vi "Begin.vi"() -> (0 "error out":errorcluster)   [LabVIEW 2013]
doc: "Called before other user functions, this VI is expected to open initial I/O refnums, load in file data, and do all program initialization. Notice that the <B>error out</B> terminal is simply used for data flow. Wiring it to other structures or subVIs ensures that this VI runs first."
uses:
  <vilib>/Rock Robotics/WPI/DriverStation/WPI_DriverStationRobotMode2.ctl
  <vilib>/Rock Robotics/WPI/Joystick/WPI_JoystickDeviceEnum.ctl
  <vilib>/Rock Robotics/SystemInterfaces/DIO/FPGA_DIOPWMChannel.ctl
  <vilib>/Rock Robotics/WPI/SafetyOutput/WPI_SafetyOutputConfigMenu.ctl
  Robot Global Data.vi
  <vilib>/Rock Robotics/WPI/RobotDrive/WPI_RobotDriveOpen4MotorWithJaguar.vi
  <vilib>/Rock Robotics/WPI/MotorControl/WPI_MotorControlOpen Jaguar.vi
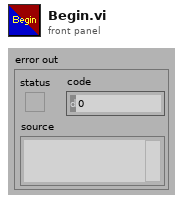
[diagram p1: front panel]
types:
  T1 = typedef "FPGA_DIOPWMChannel.ctl" = enum8{"PWM 1", "PWM 2", "PWM 3", "PWM 4", "PWM 5", "PWM 6", "PWM 7", "PWM 8", "PWM 9", "PWM 10", "Invalid"}
  T2 = typedef "WPI_SafetyOutputConfigMenu.ctl" = enum16{"Enable", "Disable"}
  T3 = typedef "WPI_JoystickDeviceEnum.ctl" = enum16{"USB 1", "USB 2", "USB 3", "USB 4", "Kinect 1", "Kinect 2"}
  T4 = typedef "WPI_DriverStationRobotMode2.ctl" = enum16{"Autonomous Disabled", "Autonomous Enabled", "Teleop Disabled", "Teleop Enabled", "Timeout", "Finish", "Test Disabled", "Test Enabled"}
  T5 = typedef "WPI_JoystickDevRef.ctl" = cluster{"Device":T3}
  T6 = typedef "WPI_MotorControlDeviceRef.ctl" = cluster{"DeviceStatus":errorcluster, "Type":enum16{"PWM", "CAN"}, "PWM":cluster{"Digital Module":T7, "PWM Channel":T1, "DeadBand":T8}, "CAN":cluster{"Device Number":u8, "Control Mode":T9, "Semaphore":T10, "Max Vout":dbl}, "Invert":bool, "TransformRef":T11, "InvTransformRef":T11}
  T7 = typedef "FPGA_TypedefDigitalModule.ctl" = enum16{"Digital Module 1", "Digital Module 2"}
  T8 = typedef "WPI_PWMDeadband.ctl" = cluster{"Name":string, "maxPositivePwm":i32, "minPositivePwm":i32, "centerPwm":i32, "maxNegativePwm":i32, "minNegativePwm":i32, "angularRange":u16}
  T9 = typedef "WPI_CANJaguar_ControlMode.ctl" = enum8{"Percent VBus", "Current", "Speed", "Position", "Voltage"}
  T10 = typedef "Semaphore RefNum" = refnum<k1>
  T11 = typedef "WPI_PWMTransform_ConPane.ctl" = refnum<vi>
  T12 = typedef "WPI_RobotDriveDevRef.ctl" = cluster{"DevStatus":errorcluster, "Motors[]":T6[], "Square Inputs":bool, "Max Output":dbl, "Isochronous":bool}
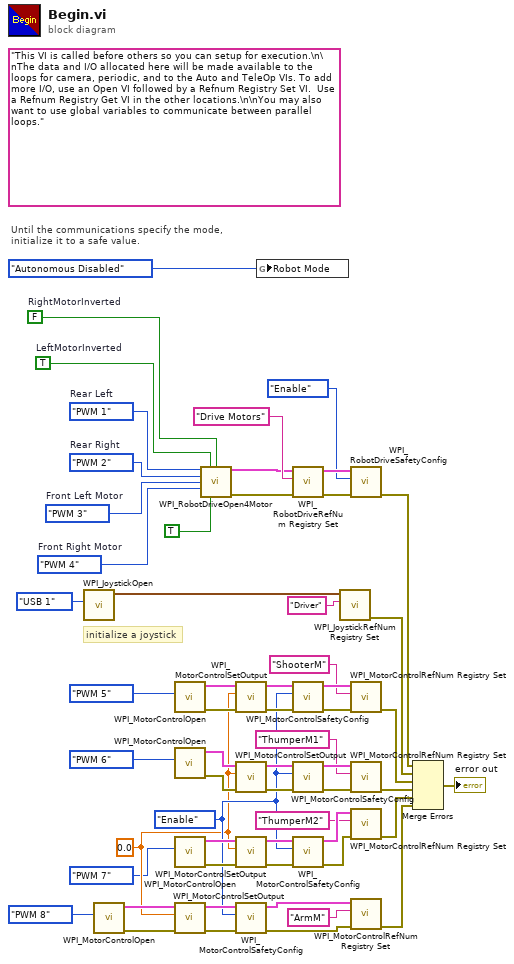
[diagram p0: block diagram]
diagram:
  w13 = 0.0 ("Output")
  w14 = WPI_SafetyOutputConfigMenu."Enable" ("mode")
  w45 = FPGA_DIOPWMChannel."PWM 4"  # Front Right Motor
  w46 = FPGA_DIOPWMChannel."PWM 3"  # Front Left Motor
  w49 = FPGA_DIOPWMChannel."PWM 2"  # Rear Right
  w50 = FPGA_DIOPWMChannel."PWM 1"  # Rear Left
  w53 = TRUE  # LeftMotorInverted
  w54 = FALSE  # RightMotorInverted
  (unwired) "This VI is called before others so you can setup for execution.\n\nThe data and I/O allocated here will be made available to the loops for camera, periodic, and to the Auto and TeleOp VIs. To add more I/O, use an Open VI followed by a Refnum Registry Set VI.  Use a Refnum Registry Get VI in the other locations.\n\nYou may also want to use global variables to communicate between parallel loops."
  # "initialize a joystick"
  # "Until the communications specify the mode,\ninitialize it to a safe value."
  n1 = call <vilib>:"WPI_JoystickOpen.vi"("JoystickDevice"=WPI_JoystickDeviceEnum."USB 1") -> ("JoystickDevRef"=w56:T5)  [unwired: 10 in]
  n2 = call-poly <vilib>:"WPI_MotorControlOpen.vi"("PWM Channel"=FPGA_DIOPWMChannel."PWM 8") -> ("error out"=w24:errorcluster, "MotorControlDeviceRef"=w25:T6)  [unwired: 9 in]
  n3 = call-poly <vilib>:"WPI_MotorControlOpen.vi"("PWM Channel"=FPGA_DIOPWMChannel."PWM 5") -> ("error out"=w15:errorcluster, "MotorControlDeviceRef"=w29:T6)  [unwired: 9 in]
  n4 = call-poly <vilib>:"WPI_MotorControlOpen.vi"("PWM Channel"=FPGA_DIOPWMChannel."PWM 6") -> ("error out"=w28:errorcluster, "MotorControlDeviceRef"=w30:T6)  [unwired: 9 in]
  n5 = call-poly <vilib>:"WPI_MotorControlOpen.vi"("PWM Channel"=FPGA_DIOPWMChannel."PWM 7") -> ("error out"=w26:errorcluster, "MotorControlDeviceRef"=w27:T6)  [unwired: 9 in]
  n6 = call <vilib>:"WPI_MotorControlSetOutput.vi"("error in (no error)"=w24, "Output"=w13, "MotorControlDevRef"=w25) -> ("error out"=w23:errorcluster, "MotorControlDevRef"=w22:T6)  [unwired: 6 in, 1 out]
  n7 = call-poly <vilib>:"WPI_RobotDriveOpen4Motor.vi"("Rear Left Motor"=w50, "Rear Left Motor Inverted"=w53, "Rear Right Motor Inverted"=w54, "Rear Right Motor"=w49, "Front Left Motor"=w46, "Front Right Motor"=w45, "Front Left Motor Inverted"=TRUE) -> ("RobotDriveDevRef"=w42:T12, "error out"=w51:errorcluster)  [unwired: 7 in]
  n8 = call <vilib>:"WPI_MotorControlSetOutput.vi"("error in (no error)"=w15, "Output"=w13, "MotorControlDevRef"=w29) -> ("error out"=w16:errorcluster, "MotorControlDevRef"=w17:T6)  [unwired: 6 in, 1 out]
  n9 = call <vilib>:"WPI_MotorControlSetOutput.vi"("error in (no error)"=w28, "Output"=w13, "MotorControlDevRef"=w30) -> ("error out"=w18:errorcluster, "MotorControlDevRef"=w19:T6)  [unwired: 6 in, 1 out]
  n10 = call <vilib>:"WPI_MotorControlSetOutput.vi"("error in (no error)"=w26, "Output"=w13, "MotorControlDevRef"=w27) -> ("error out"=w20:errorcluster, "MotorControlDevRef"=w21:T6)  [unwired: 6 in, 1 out]
  n11 = call <vilib>:"WPI_MotorControlSafetyConfig.vi"("error in (no error)"=w23, "mode"=w14, "MotorControlDevRef"=w22) -> ("error out"=w35:errorcluster, "MotorControlDevRef"=w36:T6)  [unwired: 7 in]
  n12 = global write "Robot Global Data.vi" "Robot Mode"(WPI_DriverStationRobotMode2."Autonomous Disabled" ("Robot Mode")) -> ()
  n13 = call <vilib>:"WPI_RobotDriveRefNum Registry Set.vi"("error in (no error)"=w51, "refnum name"="Drive Motors", "RobotDriveDevRef"=w42) -> ("error out"=w43:errorcluster, "RobotDriveDevRef"=w48:T12)  [unwired: 7 out]
  n14 = call <vilib>:"WPI_MotorControlSafetyConfig.vi"("error in (no error)"=w16, "mode"=w14, "MotorControlDevRef"=w17) -> ("error out"=w32:errorcluster, "MotorControlDevRef"=w33:T6)  [unwired: 7 in]
  n15 = call <vilib>:"WPI_MotorControlSafetyConfig.vi"("error in (no error)"=w18, "mode"=w14, "MotorControlDevRef"=w19) -> ("error out"=w31:errorcluster, "MotorControlDevRef"=w34:T6)  [unwired: 7 in]
  n16 = call <vilib>:"WPI_MotorControlSafetyConfig.vi"("error in (no error)"=w20, "mode"=w14, "MotorControlDevRef"=w21) -> ("error out"=w37:errorcluster, "MotorControlDevRef"=w38:T6)  [unwired: 7 in]
  n17 = call <vilib>:"WPI_JoystickRefNum Registry Set.vi"("refnum name"="Driver", "JoystickDevRef"=w56) -> ("error out"=w39:errorcluster)  [unwired: 8 in, 1 out]
  n18 = call <vilib>:"WPI_RobotDriveSafetyConfig.vi"("error in (no error)"=w43, "mode"=WPI_SafetyOutputConfigMenu."Enable", "RobotDriveDevRef"=w48) -> ("error out"=w40:errorcluster)  [unwired: 7 in, 1 out]
  n19 = call <vilib>:"WPI_MotorControlRefNum Registry Set.vi"("error in (no error)"=w32, "refnum name"="ShooterM", "MotorControlDevRef"=w33) -> ("error out"=w8:errorcluster)  [unwired: 7 in, 1 out]
  n20 = call <vilib>:"WPI_MotorControlRefNum Registry Set.vi"("error in (no error)"=w31, "refnum name"="ThumperM1", "MotorControlDevRef"=w34) -> ("error out"=w7:errorcluster)  [unwired: 7 in, 1 out]
  n21 = call <vilib>:"WPI_MotorControlRefNum Registry Set.vi"("error in (no error)"=w37, "refnum name"="ThumperM2", "MotorControlDevRef"=w38) -> ("error out"=w6:errorcluster)  [unwired: 7 in, 1 out]
  n22 = call <vilib>:"WPI_MotorControlRefNum Registry Set.vi"("error in (no error)"=w35, "refnum name"="ArmM", "MotorControlDevRef"=w36) -> ("error out"=w5:errorcluster)  [unwired: 7 in, 1 out]
  n23 = Merge Errors(w40, w39, w8, w7, w6, w5) -> (→"error out":errorcluster)
